vi "uActor_SendMsg.vi"(8 "error in (no error)":errorcluster, 10 "Msg":refnum<class "uMsg.lvclass">, 11 "uActor Transport":refnum<class "uTransport_uActor.lvclass">) -> (0 "error out":errorcluster)   [LabVIEW 2023, in "uFramework.lvlib" / "uActor.lvclass"]
doc: "Use to enqueue a request to the Actor. This is the fully fledged method that allow full messaging scalability.\n\nIt is inlined to optimize for performance but it is equivalent to the uTransport_SendMsg Method."
uses:
  uActor.lvclass
  uTransport_uActor/uTransport_uActor.lvclass
  uMsg/uMsg.lvclass
  uMsg/uMsg.lvclass/uMsg.ctl
  uTransport_uActor/uTransport_uActor.lvclass/uTransport_uActor.ctl
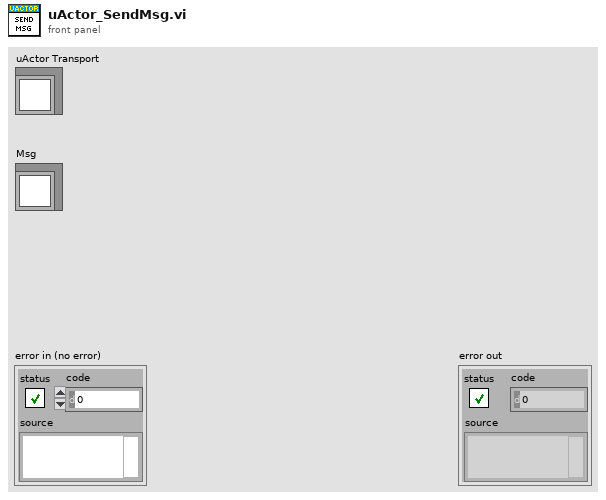
[diagram p1: front panel]
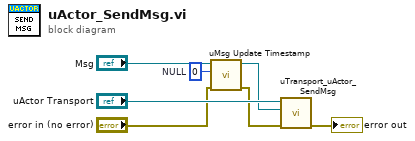
[diagram p0: block diagram]
diagram:
  w1 = u32 0  # NULL
  n1 = call "uMsg Update Timestamp.vi"("error in (no error)"="error in (no error)", "Timestamp"=w1, "uMsg in"="Msg") -> ("error out"=w3:errorcluster, "uMsg out"=w2:refnum<class "uMsg.lvclass">)  [unwired: 7 in]
  n2 = call "uTransport_uActor_SendMsg.vi"("error in (no error)"=w3, "Msg"=w2, "uTransport_uActor in"="uActor Transport") -> ("error out"=→"error out":errorcluster)  [unwired: 8 in]
